vi "poly_run_vi_path.vi"(8 "Error in":errorcluster caption="Error in (no error)", 9 "Auto dispose VI refnum?":bool=TRUE caption="Auto dispose VI refnum? (T)", 10 "Wait until VI done?":bool caption="Wait until VI done? (F)", 11 "VI path in":path) -> (0 "Error out":errorcluster, 1 "Was running?":bool, 2 "VI running?":bool, 3 "VI refnum out":refnum<vi>, 4 "Last execution state":T1(ring))   [LabVIEW 2015, in "_ref_tools_polys.lvlib"]
doc: "Runs the VI that <B>VI refnum in</B> refers to.\n\nThis function will wait until the VI is done if <B>Wait until VI done?</B> is True (default is False), and it will auto dispose the VI reference (hand it over to the running VI) if <B>Auto dispose VI refnum?</B> is True.\n\nThe VI must already be in memory (execution state \"Idle\" or \"Running\") for this function to take any action.\n\nThe <B>VI running?</B> output will only be True if the VI's <B>Last execution state</B> is \"Run top level\". Note that if this function fails to run the VI, <B>VI refnum in</B> will not be auto-disposed, in which case you retain the responsibility of closing that reference yourself.\n\nThis VI is reentrant, and it doesn't run if there is an error on <B>Error in</B>.\n\nSteen Schmidt\nGPower\n30/12 2012"
uses:
  _ref_tools_polys.lvlib
  poly_is_running_state.vi
panel:
  # "Based on Steen Schmidt, GPower"
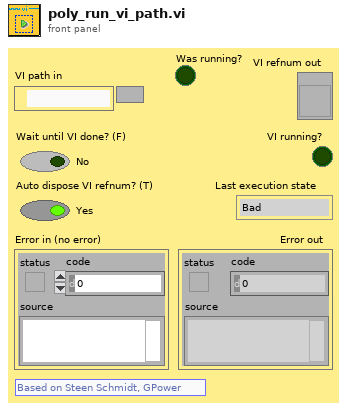
[diagram p1: front panel]
types:
  T1 = enum32{"Bad", "Idle", "Run top level", "Running"}
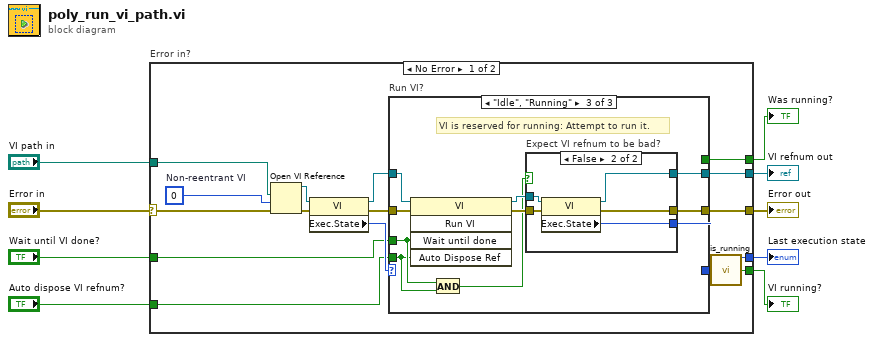
[diagram p0: block diagram]
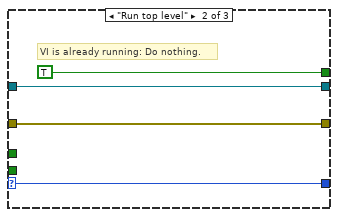
[diagram p3: hidden frame]
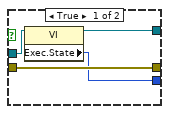
[diagram p4: hidden frame]
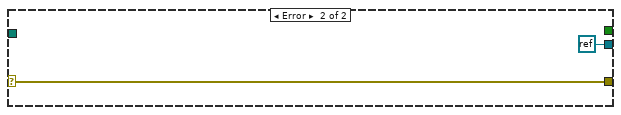
[diagram p5: hidden frame]
diagram:
  n1 = case "Error in?" shown="No Error" "Error in" {
    selector: "Error in" -> [w15 w52]
    tunnel: [w24 w52] -> w9
    tunnel: [w23 refnum<k0> refnum] -> w8
    tunnel: [w11 _] -> w7
    tunnel: [w10 _] -> w6
    tunnel: "Auto dispose VI refnum?" -> [w19 _]
    tunnel: "Wait until VI done?" -> [w18 _]
    tunnel: [w17 _] -> w3
    tunnel: "VI path in" -> [w12 _]
    frame No Error {
      w13 = 0  # Non-reentrant VI
      n2 = Open VI Reference(vi path=w12, options=w13, error in (no error)=w15) -> (vi reference=w16:refnum<vi>, error out=w14:errorcluster)  [unwired: 2 in, 1 out]
      n3 = property class="VI"(reference=w16, error in=w14) -> (reference out=w21:refnum<vi>, error out=w22:errorcluster, "Exec.State"=w20:T1)
      n4 = case "Run VI?" shown="\"Idle\", \"Running\"" w20 {
        selector: w20 -> [w25 w29 _]
        tunnel: [w27 w31 w38] -> w24
        tunnel: w22 -> [w27 w31 w41]
        tunnel: w21 -> [w26 w30 w40]
        tunnel: [w26 w30 w36] -> w23
        tunnel: [w25 w29 w35] -> w11
        tunnel: w19 -> [_ _ w33]
        tunnel: w18 -> [_ _ w34]
        tunnel: [_ TRUE _] -> w17
        frame "Bad" {
          # "VI is not in a state to be started: Do nothing."
        }
        frame "Run top level" {
          # "VI is already running: Do nothing."
        }
        frame "Idle", "Running" {
          # "VI is reserved for running: Attempt to run it."
          n5 = invoke on="Run VI" class="VI" method="Run VI"(reference=w40, error in=w41, "Wait until done"=w34, "Auto Dispose Ref"=w33) -> (reference out=w37:refnum<vi>, error out=w39:errorcluster)  [unwired: 1 in, 3 out]
          n6 = And(x=w34, y=w33) -> (x .and. y?=w32:bool)
          n7 = case "Expect VI refnum to be bad?" shown="False" w32 {
            tunnel: w39 -> [w45 w50]
            tunnel: [w45 w49] -> w38
            tunnel: w37 -> [w44 w48]
            tunnel: [w42 w47] -> w36
            tunnel: [w43 w46] -> w35
            frame True {
              n8 = property class="VI"(reference=w44) -> (reference out=w42:refnum<vi>, "Exec.State"=w43:T1)  [unwired: 1 in, 1 out]
            }
            frame False {
              n9 = property class="VI"(reference=w48, error in=w50) -> (reference out=w47:refnum<vi>, error out=w49:errorcluster, "Exec.State"=w46:T1)
            }
          }
        }
      }
      n10 = call-poly "is_running.vi"("execution state"=w11) -> ("running top level?"=w10:bool)  [unwired: 4 in]
    }
    frame Error {
    }
  }
  "Error out" <- w9
  "VI refnum out" <- w8
  "Last execution state" <- w7
  "VI running?" <- w6
  "Was running?" <- w3
